vi "Configure RemIO Module.vi"(8 "error in (no error)":errorcluster, 9 "Slave Ref In":refnum<k21>, 10 "11115 in":refnum<class "11115.lvclass">, 11 "Node Ptr In":T1 format="%.0x") -> (0 "error out":errorcluster, 1 "Slave Ref Out":refnum<k21>, 2 "11115 out":refnum<class "11115.lvclass">, 3 "Node Ptr Out":T1 format="%.0x")   [LabVIEW 2016, in "Modules.lvlib" / "11115.lvclass"]
uses:
  11115.lvclass
  <vilib>/NI Veristand/Custom Device API/Custom Device Item Ref.ctl
  11115.lvclass/11115.ctl
  <vilib>/Utility/error.llb/Error Cluster From Error Code.vi
  <vilib>/indcomecat/Remote IO/internal/_Configure REM-11115.vi
  <vilib>/ErrorRing/Error Ring.xnode
  <vilib>/indcomecat/Remote IO/NI ECAT Remote IO.lvlib
  <vilib>/NI Veristand/Custom Device API/Custom Device API.lvlib
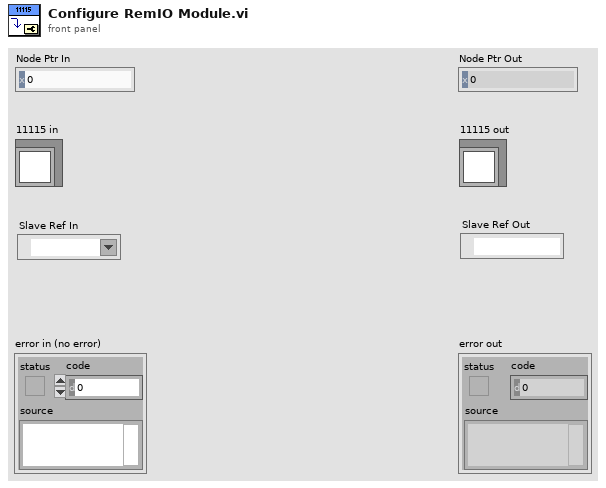
[diagram p1: front panel]
types:
  T1 = typedef "Custom Device API.lvlib/Custom Device Item Ref.ctl" = u64
  T2 = typedef "NI ECAT Remote IO.lvlib/channel number REM-11115.ctl" = u8
  T3 = typedef "NI ECAT Remote IO.lvlib/output range REM-11115.ctl" = u8
  T4 = cluster{"channel number":T2, "output range":T3}[]
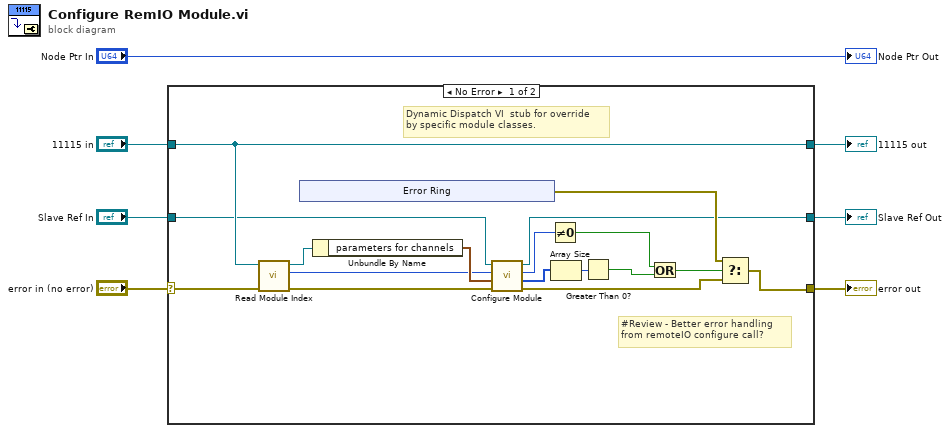
[diagram p0: block diagram]
diagram:
  n1 = case shown="No Error" "error in (no error)" {
    selector: "error in (no error)" -> [w20 w32]
    tunnel: [w21 w32] -> w6
    tunnel: [w19 w31] -> w1
    tunnel: "11115 in" -> [w19 w31]
    tunnel: [w13 w30] -> w5
    tunnel: "Slave Ref In" -> [w14 w30]
    frame No Error {
      # "#Review - Better error handling\nfrom remoteIO configure call?"
      # "Dynamic Dispatch VI  stub for override\nby specific module classes."
      n2 = call-dynamic "Read Module Index.vi"("error in (no error)"=w20, "RemIO Module in"=w19) -> ("error out"=w16:errorcluster, "Module Index"=w8:u8, "RemIO Module out"=w10:refnum<class "11115.lvclass">)  [unwired: 7 in]
      n3 = xnode "Error Ring"() -> ("error out"=w22:errorcluster)
      n4 = Unbundle By Name(w10) -> ("parameters for channels"=w9:T4)
      n5 = call-poly <vilib>:"Configure Module.vi"("error in (no error)"=w16, "parameters for channels"=w9, "module slot index"=w8, "slave reference in"=w14) -> ("error out"=w15:errorcluster, "negative confirmation"=w12:u8[], "SDO abort code"=w11:u32, "slave reference out"=w13:refnum<k21>)  [unwired: 4 in]
      n6 = Not Equal To 0?(x=w11) -> (x != 0?=w17:bool)
      n7 = Array Size(array=w12) -> (size(s)=w24:i32)
      n8 = Greater Than 0?(x=w24) -> (x > 0?=w23:bool)
      n9 = Or(x=w17, y=w23) -> (x .or. y?=w18:bool)
      n10 = Select(t=w22, s=w18, f=w15) -> (s? t:f=w21:errorcluster)
    }
    frame Error {
    }
  }
  "error out" <- w6
  "11115 out" <- w1
  "Slave Ref Out" <- w5
  "Node Ptr Out" <- "Node Ptr In"
